vi "FLL Tournament Display Double Qualifier.vi"() -> ()   [LabVIEW 2013]
uses:
  Team_List_Ctrl.ctl
  Team_Scores_And_Rankings_Array_Ctrl.ctl
  Round_And_Score_Ctrl.ctl
  Timer_Details_Ctrl.ctl
  Sound Info.ctl
  <vilib>/sound2/lvsound2.llb/Sound Data Format.ctl
  <vilib>/sound2/lvsound2.llb/Sampling Mode.ctl
  SponsorImageFreqArray.ctl
  <vilib>/picture/picture.llb/imagedata.ctl
  <vilib>/sound2/lvsound2.llb/Sound Output Set Volume (Single).vi
  <vilib>/sound2/lvsound2.llb/Sound Output Write (DBL).vi
  <vilib>/httpClient/LabVIEWHTTPClient.lvlib
panel:
  out "SFA 2":string[][](array[string])
  out "Full Team List 2":T1[](array[typedef])
  out "Reported Scores and Rankings 2":T2
  out "Consolidated Scores and Rankings 2":T4(array[cluster])
  out "IP Address / Port 2":string
  in  "Hurry-Up Sound Volume":dbl(slide)=88.46153846153847 scale=0.0..100.0
  in  "Pre-Match Coundown Sound Volume":dbl(slide)=88.46153846153847 scale=0.0..100.0
  in  "Uh-Oh Sound Volume":dbl(slide)=88.46153846153847 scale=0.0..100.0
  in  "Stop Sound Volume":dbl(slide)=100.0 scale=0.0..100.0
  in  "Start Sound Volume":dbl(slide)=100.0 scale=0.0..100.0
  out "Sound Cluster 2":T5={"Start"={"total number of samples/ch"=31680, "sound format"={"sample rate (S/s)"=11025.0, "number of channels"=1, "bits per sample"=16}, "data"=[{"t0"=timestamp(0 s since 1904-01-01), "dt"=9.070294784580499e-05, "Y"=array[31680 elements]}], "Volume"=100.0}, "Stop"={"total number of samples/ch"=27648, "sound format"={"sample rate (S/s)"=11025.0, "number of channels"=1, "bits per sample"=16}, "data"=[{"t0"=timestamp(0 s since 1904-01-01), "dt"=9.070294784580499e-05, "Y"=array[27648 elements]}], "Volume"=100.0}, "Uh-Oh"={"total number of samples/ch"=29952, "sound format"={"sample rate (S/s)"=11025.0, "number of channels"=1, "bits per sample"=16}, "data"=[{"t0"=timestamp(0 s since 1904-01-01), "dt"=9.070294784580499e-05, "Y"=array[29952 elements]}], "Volume"=88.46153846153847}, "PreMatch"={"total number of samples/ch"=225792, "sound format"={"sample rate (S/s)"=44100.0, "number of channels"=2, "bits per sample"=16}, "data"=[{"t0"=timestamp(0 s since 1904-01-01), "dt"=2.2675736961451248e-05, "Y"=array[225792 elements]}, {"t0"=timestamp(0 s since 1904-01-01), "dt"=2.2675736961451248e-05, "Y"=array[225792 elements]}], "Volume"=75.38461538461539}, "Hurry-Up"={"total number of samples/ch"=0, "sound format"={"sample rate (S/s)"=0.0, "number of channels"=0, "bits per sample"=0}, "data"=[], "Volume"=0.0}}
  in  "stop":bool
  in  "Sound To Play":T7(ring)
  out "Primary Sound Array":dbl[](array[numeric])
  out "PrePrimary Sound Array":dbl[](array[numeric])
  out "Secondary (s)":dbl
  out "Primary (s)":dbl
  out "Pre-Primary (s)":dbl
  out "Master Volume":dbl
  out "Sound Cluster":T5={"Start"={"total number of samples/ch"=31680, "sound format"={"sample rate (S/s)"=11025.0, "number of channels"=1, "bits per sample"=16}, "data"=[{"t0"=timestamp(0 s since 1904-01-01), "dt"=9.070294784580499e-05, "Y"=array[31680 elements]}], "Volume"=100.0}, "Stop"={"total number of samples/ch"=27648, "sound format"={"sample rate (S/s)"=11025.0, "number of channels"=1, "bits per sample"=16}, "data"=[{"t0"=timestamp(0 s since 1904-01-01), "dt"=9.070294784580499e-05, "Y"=array[27648 elements]}], "Volume"=100.0}, "Uh-Oh"={"total number of samples/ch"=29952, "sound format"={"sample rate (S/s)"=11025.0, "number of channels"=1, "bits per sample"=16}, "data"=[{"t0"=timestamp(0 s since 1904-01-01), "dt"=9.070294784580499e-05, "Y"=array[29952 elements]}], "Volume"=88.46153846153847}, "PreMatch"={"total number of samples/ch"=225792, "sound format"={"sample rate (S/s)"=44100.0, "number of channels"=2, "bits per sample"=16}, "data"=[{"t0"=timestamp(0 s since 1904-01-01), "dt"=2.2675736961451248e-05, "Y"=array[225792 elements]}, {"t0"=timestamp(0 s since 1904-01-01), "dt"=2.2675736961451248e-05, "Y"=array[225792 elements]}], "Volume"=75.38461538461539}, "Hurry-Up"={"total number of samples/ch"=0, "sound format"={"sample rate (S/s)"=0.0, "number of channels"=0, "bits per sample"=0}, "data"=[], "Volume"=0.0}}
  out "EnableSounds":bool
  out "Score Behavior":T8(ring)
  out "SFA":string[][](array[string])
  out "NumRoundsToShow":string
  out "Cancelled?":bool
  out "IP Address / Port":string
  in  "Scores Tab":enum32{"3 Rounds", "4 Rounds"}(tab)
  out "Division 1 String 2":string="TESLA DIVISION"
  in  "Scores Box 3":i32[](listbox)
  out "Division 1 String":string="LOVELACE DIVISION"
  in  "Scores Box":i32[](listbox)
  in  "Scores Box 2":i32(listbox)=3
  in  "Top Tab":enum32{"Page 1"}(tab)
  out "Main Logo Image":picture
  out "Powered By LabVIEW":picture
  out "FIRST LEGO League":picture
  out "Match Indicator":string
  out "Tournament Title String":string="Central Texas FLL - Del Valle Double Qualifier Tournament"
  out "TIMER":string="2 : 3 0"
  out "Top Sponsor Image":picture
  out "Mid Sponsor Image":picture
  out "Bottom Sponsor Image":picture
  out "Timer Properties":T9
  out "Consolidated Scores and Rankings":T4(array[cluster])
  out "Reported Scores and Rankings":T2
  out "Full Team List":T1[](array[typedef])
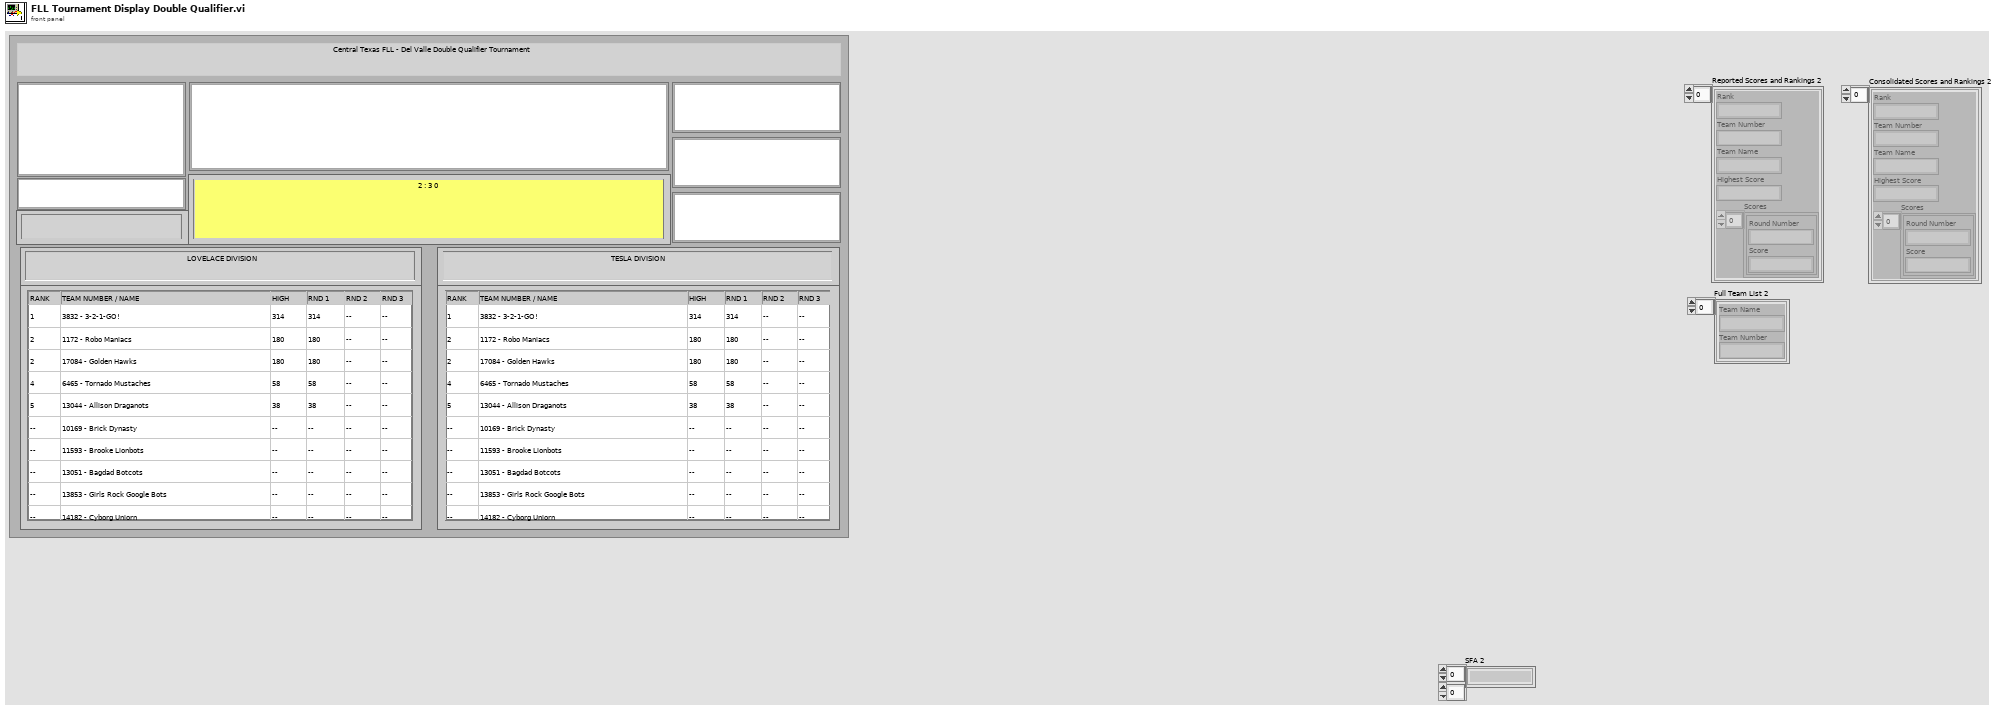
[diagram p1: front panel]
types:
  T1 = typedef "Team_List_Ctrl.ctl" = cluster{"Team Name":string, "Team Number":string}
  T2 = typedef "Team_Scores_And_Rankings_Array_Ctrl.ctl" = cluster{"Rank":string, "Team Number":string, "Team Name":string, "Highest Score":string, "Scores":T3[]}[]
  T3 = typedef "Round_And_Score_Ctrl.ctl" = cluster{"Score":string, "Round Number":string}
  T4 = cluster{"Rank":string, "Team Number":string, "Team Name":string, "Highest Score":string, "Scores":T3[]}[]
  T5 = typedef "Sound Info.ctl" = cluster{"Start":cluster{"total number of samples/ch":u32, "sound format":T6, "data":waveform(dbl)[], "Volume":dbl}, "Stop":cluster{"total number of samples/ch":u32, "sound format":T6, "data":waveform(dbl)[], "Volume":dbl}, "Uh-Oh":cluster{"total number of samples/ch":u32, "sound format":T6, "data":waveform(dbl)[], "Volume":dbl}, "PreMatch":cluster{"total number of samples/ch":u32, "sound format":T6, "data":waveform(dbl)[], "Volume":dbl}, "Hurry-Up":cluster{"total number of samples/ch":u32, "sound format":T6, "data":waveform(dbl)[], "Volume":dbl}}
  T6 = typedef "Sound Data Format.ctl" = cluster{"sample rate (S/s)":dbl, "number of channels":i32, "bits per sample":i32}
  T7 = enum16{"None", "Start", "Stop", "Uh-Oh", "Prematch", "Hurry-Up"}
  T8 = enum16{"Show Negative Scores as ZERO", "Show Negative Scores"}
  T9 = typedef "Timer_Details_Ctrl.ctl" = cluster{"TimeRemaining":string, "MatchPhase":string, "CurrentMatch":string, "Timer_Running":string, "Seconds":string, "LastSound":string}
  T10 = cluster{"Master Volume":dbl, "Pre-Primary (s)":dbl, "Primary (s)":dbl, "Secondary (s)":dbl, "Start Sound Path":path, "Stop Sound Path":path, "Uh-Oh Sound Path":path, "Pre-Match Countdown Sound":path, "Hurry Up Sound":path, "Start Sound Volume":dbl, "Stop Sound Volume":dbl, "Uh-Oh Sound Volume":dbl, "Pre-Match Coundown Sound Volume":dbl, "Hurry Up Sound Volume":dbl}
  T11 = typedef "SponsorImageFreqArray.ctl" = cluster{"Cluster":cluster{"Array":T12[], "Frequency (s)":dbl}, "Cluster":cluster{"Array":T12[], "Frequency (s)":dbl}, "Cluster":cluster{"Array":T12[], "Frequency (s)":dbl}}
  T12 = typedef "imagedata.ctl" = cluster{"image type":i32, "image depth":i32, "image":u8[], "mask":u8[], "colors":u32[], "Rectangle":cluster{"left":i16, "top":i16, "right":i16, "bottom":i16}}
  T13 = typedef "LabVIEWHTTPClient.lvlib/ClientHandle.ctl" = refnum<k1>
  T14 = typedef "Team_List_Array_Ctrl.ctl" = T1[]
  T15 = cluster{"[0]":string, "[1]":string, "[2]":string, "[3]":string}
  T16 = enum32{"Invalid", "Standard", "Closed", "Hidden", "Minimized", "Maximized"}
  T17 = enum32{"invalid app kind", "Development System", "Run Time System", "Student Edition", "Embedded LabVIEW", "Evaluation", "Custom"}
  T18 = cluster{"total number of samples/ch":u32, "sound format":T6, "data":waveform(dbl)[], "Volume":dbl}
  T19 = typedef "Sampling Mode.ctl" = i32
  T20 = typedef "Sound Output Task ID.ctl" = u32
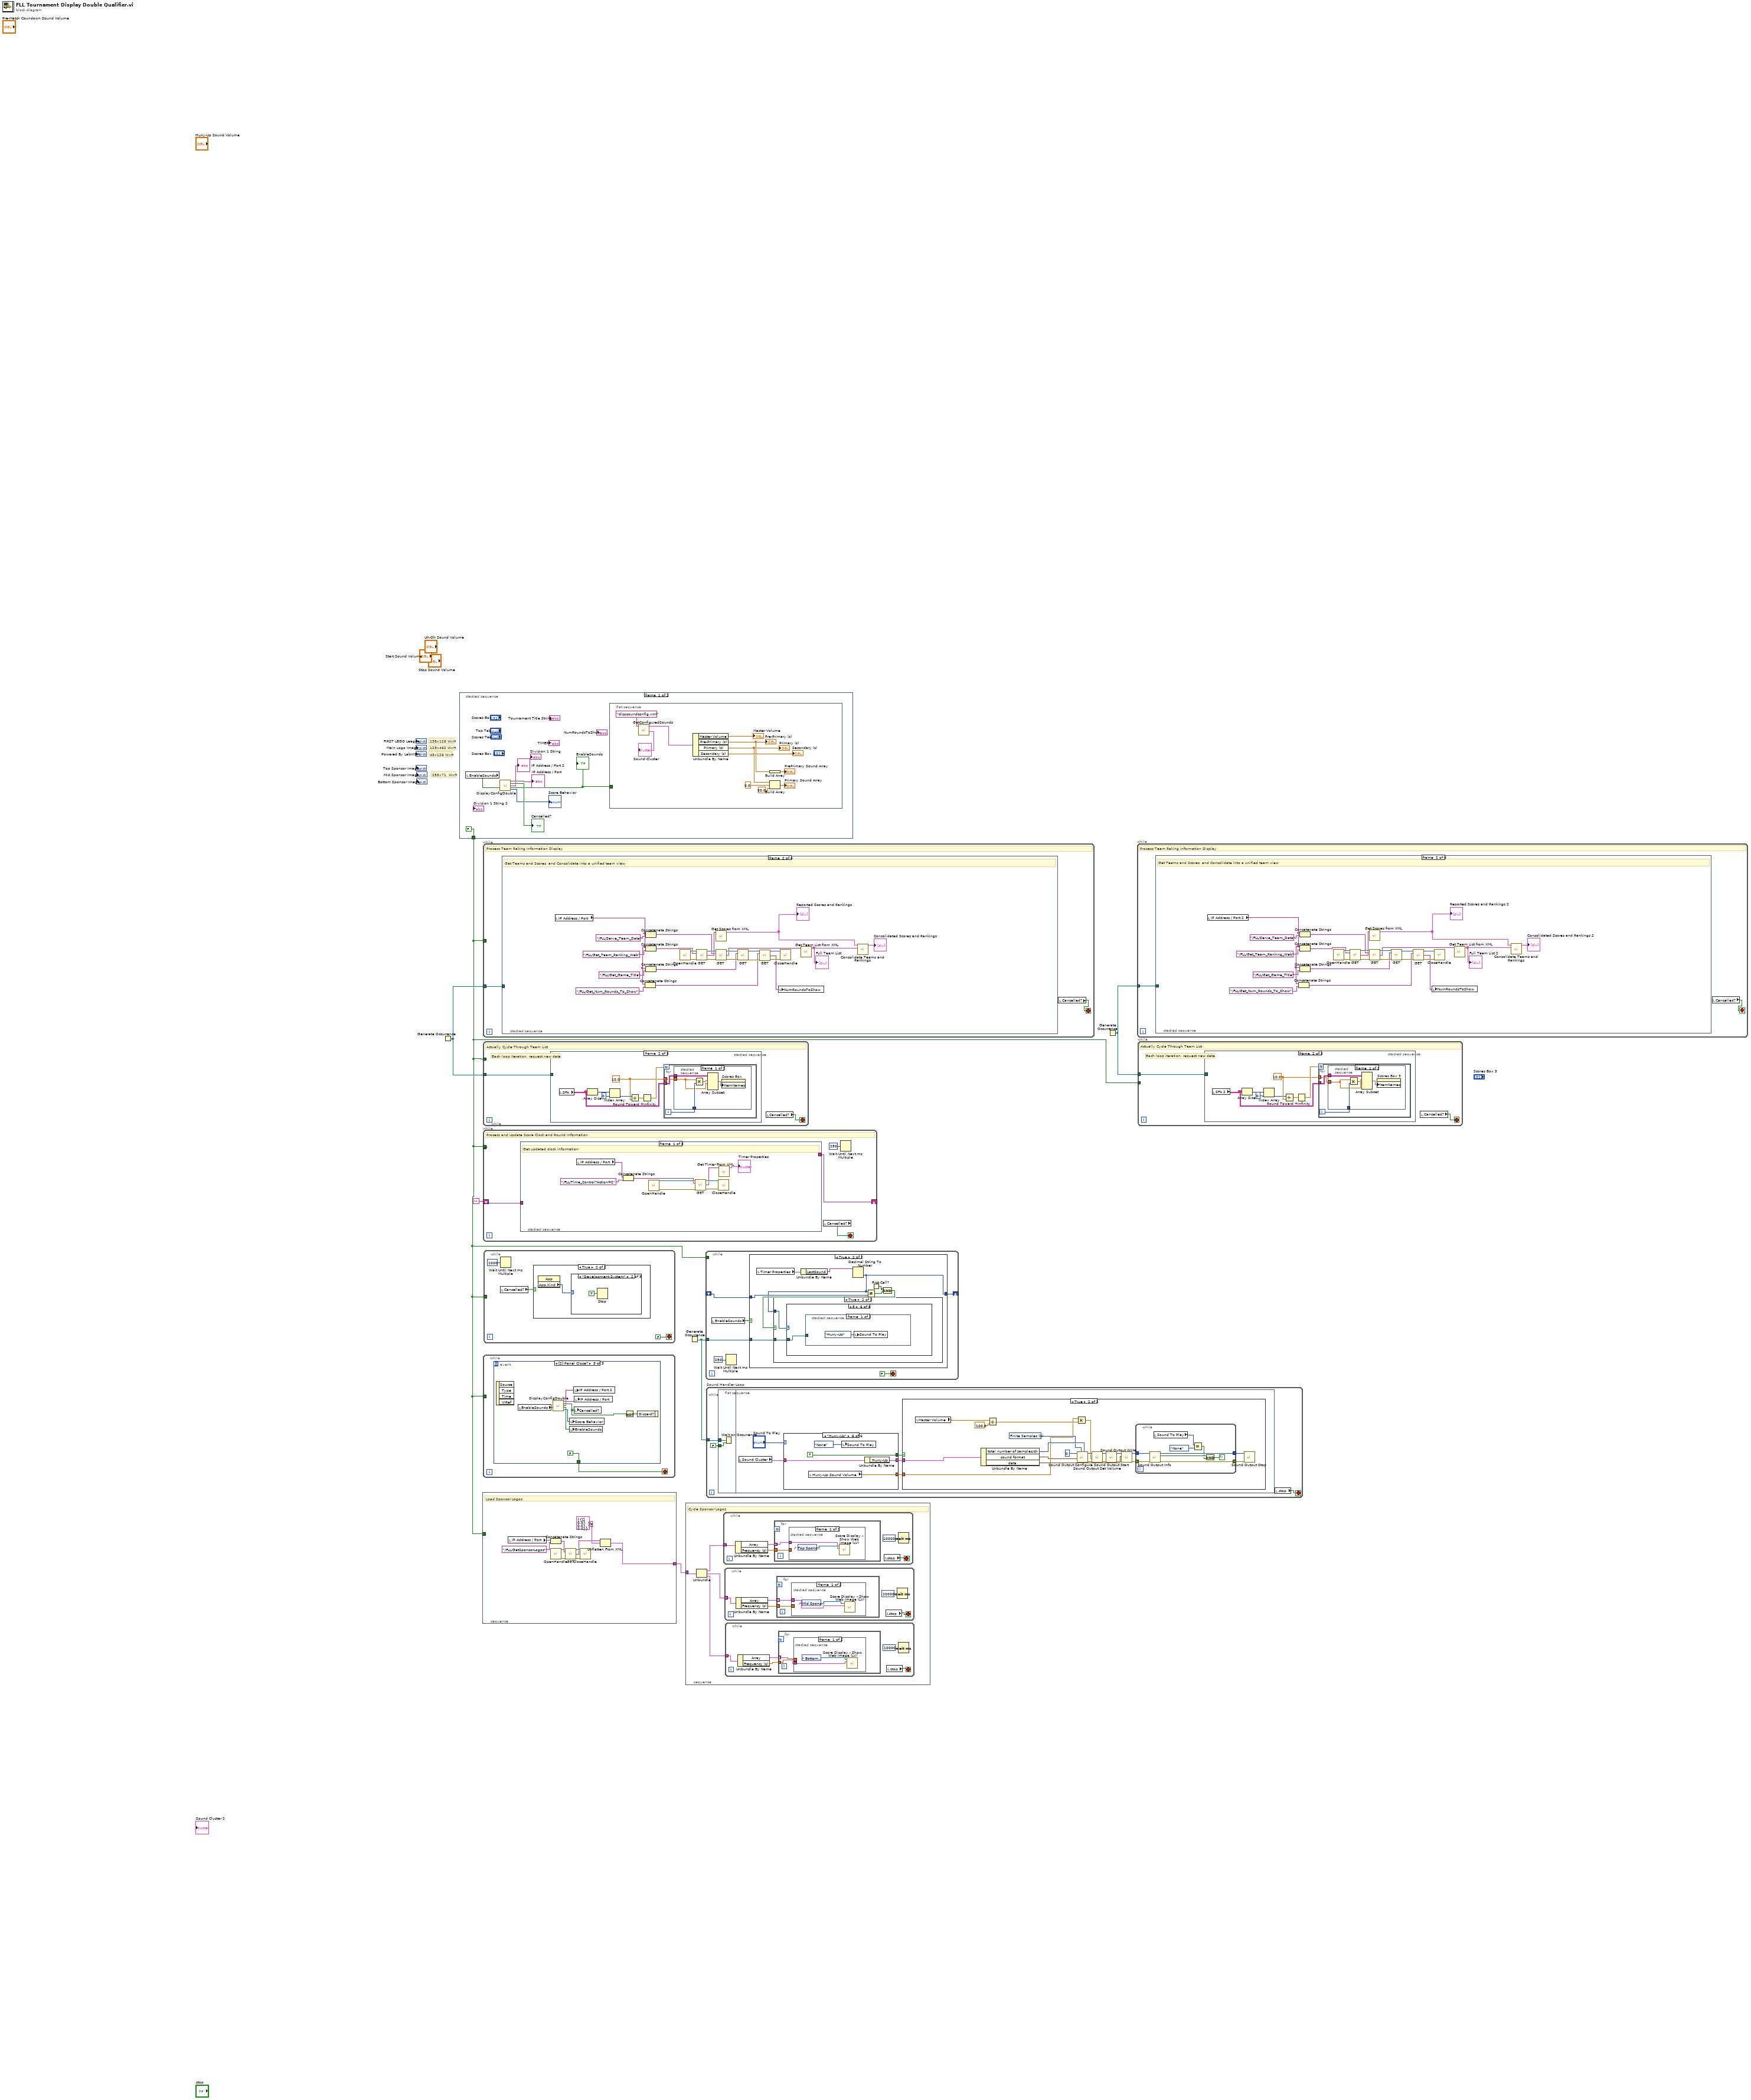
[diagram p0: block diagram]
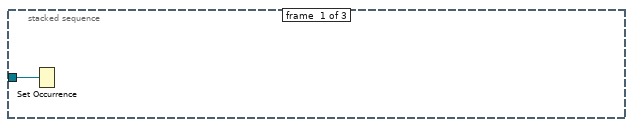
[diagram p2: hidden frame]
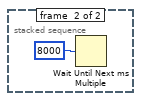
[diagram p3: hidden frame]
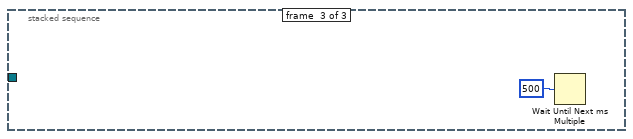
[diagram p4: hidden frame]
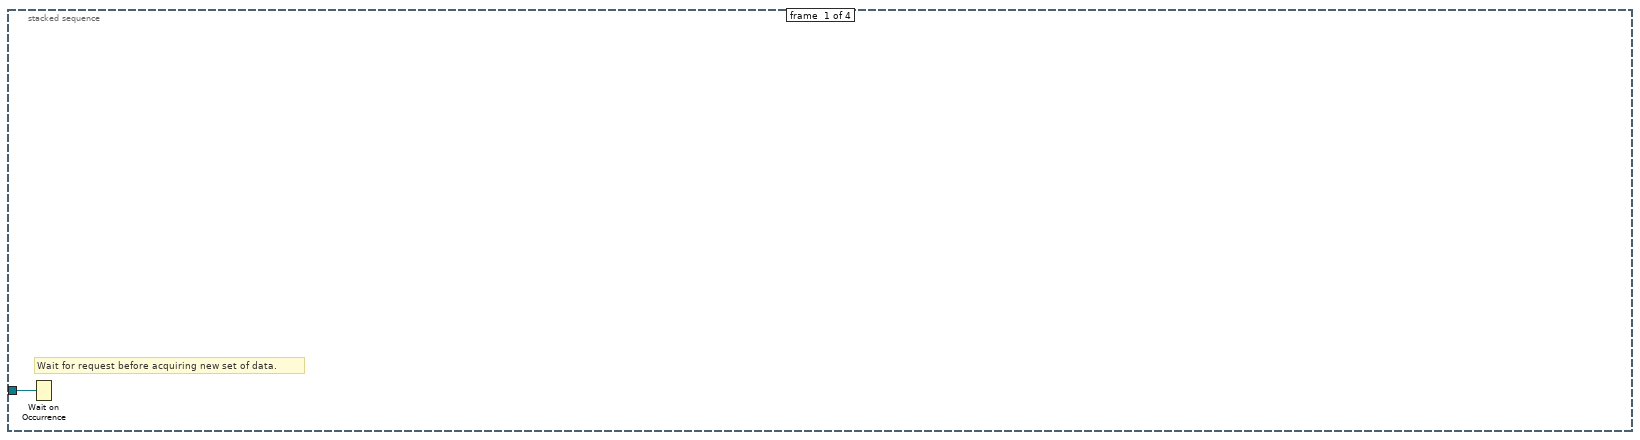
[diagram p5: hidden frame]
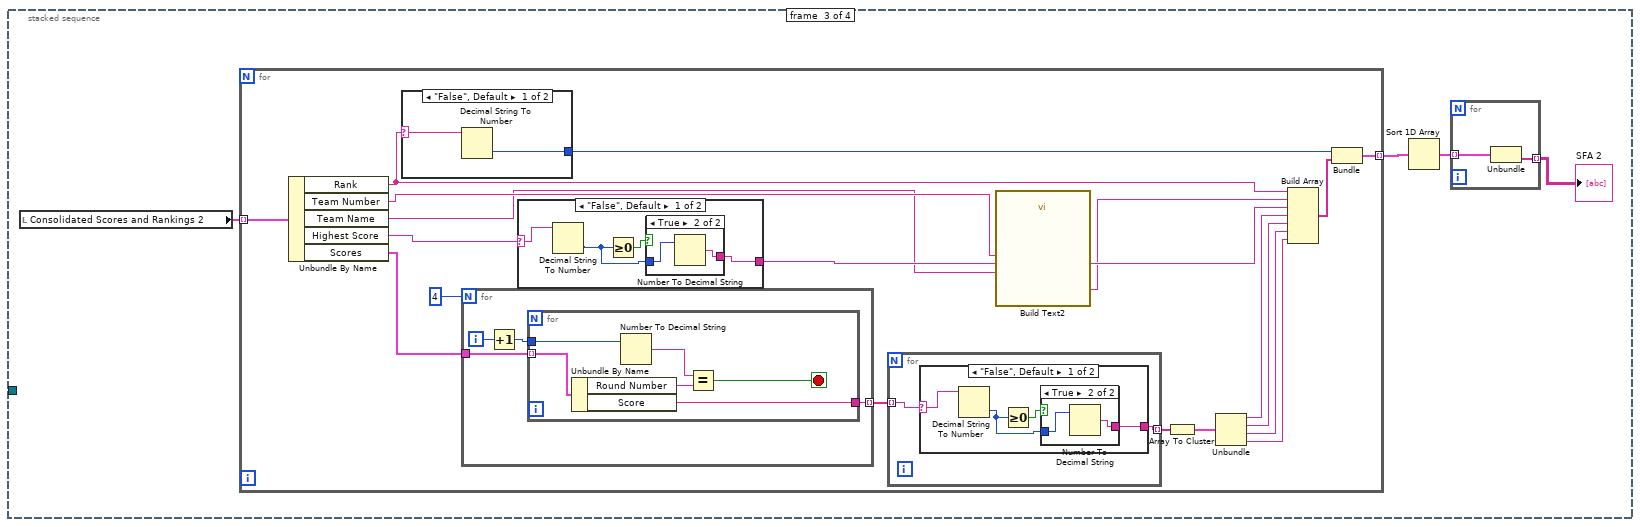
[diagram p6: hidden frame]
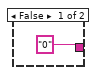
[diagram p7: hidden frame]
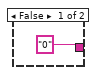
[diagram p9: hidden frame]
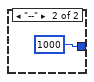
[diagram p11: hidden frame]
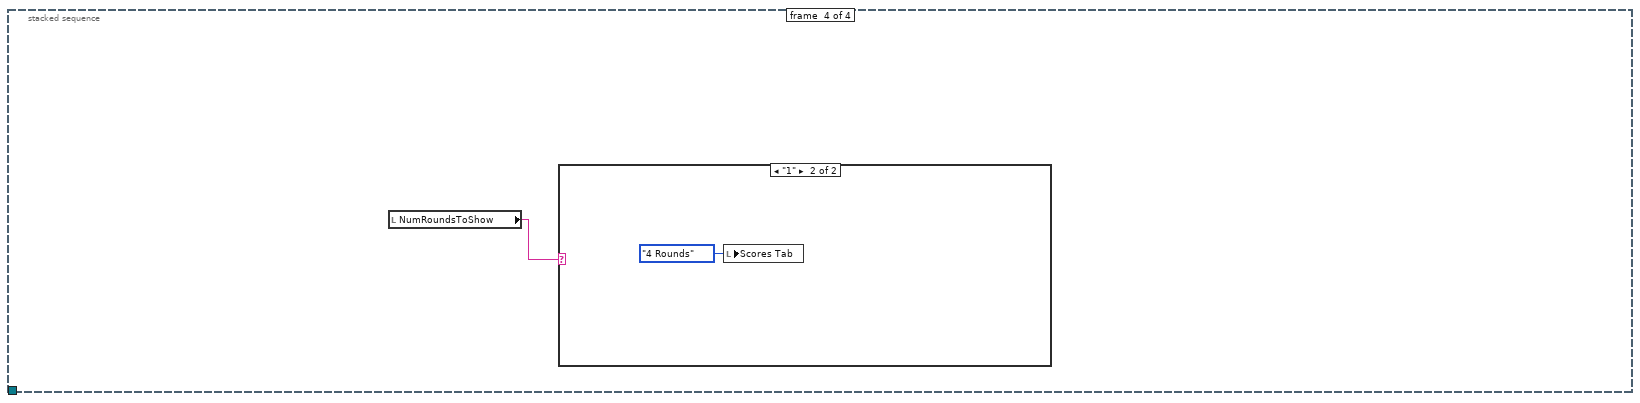
[diagram p12: hidden frame]
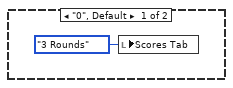
[diagram p13: hidden frame]
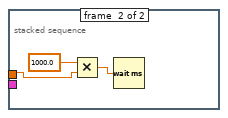
[diagram p14: hidden frame]
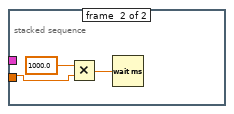
[diagram p15: hidden frame]
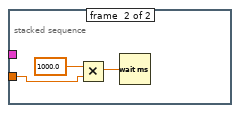
[diagram p16: hidden frame]
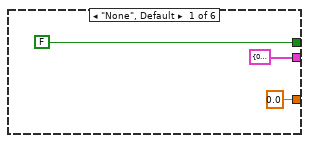
[diagram p18: hidden frame]
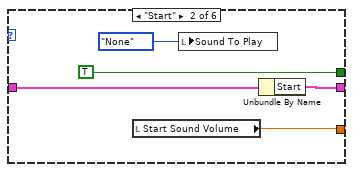
[diagram p19: hidden frame]
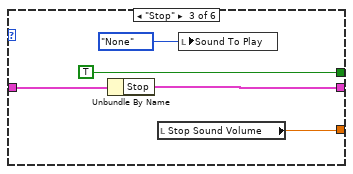
[diagram p20: hidden frame]
diagram:
  # "129x462 WxH"
  # "43x126 WxH"
  # "253x71  WxH"
  # "138x126 WxH"
  n1 = Generate Occurrence() -> (w5:refnum<k4>)
  n2 = stacked-sequence {
    tunnel: [FALSE _] -> w1
    frame #0 {
      n3 = local read "EnableSounds"() -> (w9:bool)
      n4 = call "DisplayConfigDouble.vi"("EnableSounds"=w9) -> ("LovelaceIP"=→"IP Address / Port":string, "Cancelled?"=→"Cancelled?":bool, "TeslaIP"=→"IP Address / Port 2":string, "EnableSounds out"=w8:bool, "Score Behavior OUT"=→"Score Behavior":T8)  [unwired: 10 in]
      "EnableSounds" <- w8
      n5 = flat-sequence {
        tunnel: w8 -> [_]
        frame #0 {
          n6 = call "GetConfiguredSounds.vi"("File"="dispsoundconfig.xml") -> ("Sound Cluster"=→"Sound Cluster":T5, "Settings Cluster"=w23:T10)  [unwired: 9 in]
          n7 = Unbundle By Name(w23) -> ("Master Volume"=→"Master Volume":dbl, "Pre-Primary (s)"=w20:dbl, "Primary (s)"=w18:dbl, "Secondary (s)"=→"Secondary (s)":dbl)
          "Pre-Primary (s)" <- w20
          "Primary (s)" <- w18
          n8 = Build Array(w20) -> (→"PrePrimary Sound Array":dbl[])
          n9 = Build Array(w18, 0.0 ("element"), 30.0 ("element")) -> (→"Primary Sound Array":dbl[])
        }
      }
    }
    frame #1 {
      n10 = disable-structure shown="Disabled" {
        frame Disabled {
          n11 = control-ref of="Powered By LabVIEW"() -> (w29:refnum<vi>)
          n12 = call "Score Display - Auto Scale Image (LV).vi"("Picture Reference"=w29, "path to image file"=path "C:/Users/Danny Diaz/Dropbox/FLL 2 (1).1/Images/powered-by-labview-horiz-logo-rgb.png") -> ()  [unwired: 1 out]
        }
        frame Enabled {
        }
      }
      n13 = disable-structure shown="Disabled" {
        frame Disabled {
          n14 = control-ref of="FIRST LEGO League"() -> (w27:refnum<vi>)
          n15 = call "Score Display - Auto Scale Image (LV).vi"("Picture Reference"=w27, "path to image file"=path "C:/Users/Danny Diaz/Dropbox/FLL 2 (1).1/Images/FLLicon_RGB.jpg") -> ()  [unwired: 1 out]
        }
        frame Enabled {
        }
      }
      n16 = disable-structure shown="Disabled" {
        frame Disabled {
          n17 = control-ref of="Main Logo Image"() -> (w25:refnum<vi>)
          n18 = call "Score Display - Auto Scale Image (LV).vi"("Picture Reference"=w25, "path to image file"=path "C:/Users/Danny Diaz/Dropbox/FLL 2 (1).1/Images/res Fury Logo SM.jpg") -> ()  [unwired: 1 out]
        }
        frame Enabled {
        }
      }
    }
  }
  n19 = stacked-sequence {
    tunnel: w1 -> [_]
    tunnel: [w31] -> w4
    frame #0 {
      # "Load Sponsor Logos"
      n20 = local read "IP Address / Port"() -> (w40:string)
      n21 = Concatenate Strings(w40, "/FLL/GetSponsorLogos" ("url")) -> (w39:string)
      n22 = call <vilib>:"OpenHandle.vi"() -> ("client handle out"=w35:T13, "error out"=w34:errorcluster)  [unwired: 14 in]
      n23 = call <vilib>:"GET.vi"("client handle"=w35, "url"=w39, "error in (no error)"=w34) -> ("client handle out"=w36:T13, "body"=w33:string, "error out"=w37:errorcluster)  [unwired: 9 in, 1 out]
      n24 = call <vilib>:"CloseHandle.vi"("client handle"=w36, "error in (no error)"=w37) -> ()  [unwired: 13 in, 1 out]
      n25 = Unflatten From XML(xml string=w33, type=T11 {"Cluster"={"Array"=[], "Frequency (s)"=0.0}, "Cluster"={"Array"=[], "Frequency (s)"=0.0}, "Cluster"={"Array"=[], "Frequency (s)"=0.0}} ("output cluster")) -> (value=w31:T11)  [unwired: 1 in, 1 out]
    }
  }
  n26 = while {
    tunnel: w1 -> [_]
    tunnel: w5 -> [w41]
    stop <- w42 stop-if-true
    # "Process Team Raking Information Display"
    n27 = stacked-sequence {
      tunnel: w41 -> [w43 _ _ _]
      frame #0 {
        # "Wait for request before acquiring new set of data."
        n28 = Wait on Occurrence(2:w43) -> ()  [unwired: 2 in, 1 out]
      }
      frame #1 {
        # "Get Teams and Scores, and Consolidate into a unified team view"
        n29 = local read "IP Address / Port"() -> (w46:string)
        n30 = Concatenate Strings(w46, "/FLL/Get_Num_Rounds_To_Show" ("url")) -> (w45:string)
        n31 = Concatenate Strings(w46, "/FLL/Serve_Team_Data" ("url")) -> (w59:string)
        n32 = Concatenate Strings(w46, "/FLL/Get_Team_Ranking_Web" ("url")) -> (w57:string)
        n33 = Concatenate Strings(w46, "/FLL/Get_Game_Title" ("url")) -> (w52:string)
        n34 = call <vilib>:"OpenHandle.vi"() -> ("client handle out"=w68:T13, "error out"=w66:errorcluster)  [unwired: 14 in]
        n35 = call <vilib>:"GET.vi"("client handle"=w68, "url"=w57, "error in (no error)"=w66) -> ("client handle out"=w65:T13, "body"=w64:string, "error out"=w67:errorcluster)  [unwired: 9 in, 1 out]
        n36 = call "Get Scores from XML.vi"("XML In"=w64) -> ("Team_Scores_And_Rankings_Array"=w62:T4)  [unwired: 10 in]
        "Reported Scores and Rankings" <- w62
        n37 = call <vilib>:"GET.vi"("client handle"=w65, "url"=w59, "error in (no error)"=w67) -> ("client handle out"=w56:T13, "body"=w54:string, "error out"=w55:errorcluster)  [unwired: 9 in, 1 out]
        n38 = call <vilib>:"GET.vi"("client handle"=w56, "url"=w52, "error in (no error)"=w55) -> ("client handle out"=w48:T13, "error out"=w49:errorcluster)  [unwired: 9 in, 2 out]
        n39 = call <vilib>:"GET.vi"("client handle"=w48, "url"=w45, "error in (no error)"=w49) -> ("client handle out"=w51:T13, "body"=w44:string, "error out"=w50:errorcluster)  [unwired: 9 in, 1 out]
        n40 = local write "NumRoundsToShow"(w44) -> ()
        n41 = call <vilib>:"CloseHandle.vi"("client handle"=w51, "error in (no error)"=w50) -> ()  [unwired: 13 in, 1 out]
        n42 = call "Get Team List from XML.vi"("XML In"=w54) -> ("Team List Array"=w63:T14)  [unwired: 10 in]
        "Full Team List" <- w63
        n43 = call "Consolidate Teams and Rankings.vi"("Team List Array"=w63, "Team_Scores_And_Rankings_Array"=w62) -> ("Consolidated Teams and Rankings"=→"Consolidated Scores and Rankings":T4)  [unwired: 9 in]
      }
      frame #2 {
        n44 = local read "Consolidated Scores and Rankings"() -> (w72:T4)
        n45 = for {
          tunnel: w72 -> [w83] mode=indexing
          tunnel: [w82] -> w70 mode=indexing
          n46 = Unbundle By Name(w83) -> ("Rank"=w85:string, "Team Number"=w77:string, "Team Name"=w76:string, "Highest Score"=w81:string, "Scores"=w93:T3[])
          n47 = case shown="\"False\", Default" w85 {
            selector: w85 -> [w113 _]
            tunnel: [w112 1000] -> w84
            frame "False", Default {
              n48 = Decimal String To Number(string=w113) -> (number=w112:i32)  [unwired: 2 in, 1 out]
            }
            frame "--" {
            }
          }
          n49 = for {
            N: 4 -> [_]
            tunnel: w93 -> [w117]
            tunnel: [w115] -> w79 mode=indexing
            i -> [w118]
            n50 = Increment(x=w118) -> (x+1=w116:i32)
            n51 = for {
              tunnel: w117 -> [w120] mode=indexing
              tunnel: w116 -> [w124]
              tunnel: [w119] -> w115
              stop <- w121 stop-if-true
              n52 = Unbundle By Name(w120) -> ("Round Number"=w123:string, "Score"=w119:string)
              n53 = Number To Decimal String(number=w124) -> (decimal integer string=w122:string)  [unwired: 1 in]
              n54 = Equal?(x=w122, y=w123) -> (x = y?=w121:bool)
            }
          }
          n55 = case shown="\"False\", Default" w81 {
            selector: w81 -> [w107 w111]
            tunnel: [w105 w111] -> w80
            frame "False", Default {
              n56 = Decimal String To Number(string=w107) -> (number=w104:i32)  [unwired: 2 in, 1 out]
              n57 = Greater Or Equal To 0?(x=w104) -> (x >= 0?=w106:bool)
              n58 = case shown="True" w106 {
                tunnel: ["0" w110] -> w105
                tunnel: w104 -> [_ w109]
                frame False {
                }
                frame True {
                  n59 = Number To Decimal String(number=w109) -> (decimal integer string=w110:string)  [unwired: 1 in]
                }
              }
            }
            frame "--" {
            }
          }
          n60 = for {
            tunnel: w79 -> [w95] mode=indexing
            tunnel: [w94] -> w78 mode=indexing
            n61 = case shown="\"False\", Default" w95 {
              selector: w95 -> [w98 w103]
              tunnel: [w99 w103] -> w94
              frame "False", Default {
                n62 = Decimal String To Number(string=w98) -> (number=w96:i32)  [unwired: 2 in, 1 out]
                n63 = Greater Or Equal To 0?(x=w96) -> (x >= 0?=w97:bool)
                n64 = case shown="True" w97 {
                  tunnel: ["0" w102] -> w99
                  tunnel: w96 -> [_ w101]
                  frame False {
                  }
                  frame True {
                    n65 = Number To Decimal String(number=w101) -> (decimal integer string=w102:string)  [unwired: 1 in]
                  }
                }
              }
              frame "--" {
              }
            }
          }
          n66 = call "Build Text"("team_number"=w77, "team_name"=w76) -> ("Result"=w75:string)  [unwired: 12 in, 1 out]
          n67 = Array To Cluster(array=w78) -> (cluster=w91:T15)
          n68 = Unbundle(w91) -> ("[0]"=w90:string, "[1]"=w89:string, "[2]"=w88:string, "[3]"=w87:string)
          n69 = Build Array(w85, w75, w80, w90, w89, w88, w87) -> (w86:string[])
          n70 = Bundle(w84, w86) -> (w82:cluster{i32, string[]})  [unwired: 1 in]
        }
        n71 = Sort 1D Array(array=w70) -> (sorted array=w71:cluster{i32, string[]}[])
        n72 = for {
          tunnel: w71 -> [w74] mode=indexing
          tunnel: [w73] -> w69 mode=indexing
          n73 = Unbundle(w74) -> (w73:string[])  [unwired: 1 out]
        }
        "SFA" <- w69
      }
      frame #3 {
        n74 = local read "NumRoundsToShow"() -> (w125:string)
        n75 = case shown="\"1\"" w125 {
          frame "0", Default {
            n76 = local write "Scores Tab"(enum32{"3 Rounds", "4 Rounds"}."3 Rounds" ("Scores Tab")) -> ()
          }
          frame "1" {
            n77 = local write "Scores Tab"(enum32{"3 Rounds", "4 Rounds"}."4 Rounds" ("Scores Tab")) -> ()
          }
        }
      }
    }
    n78 = local read "Cancelled?"() -> (w42:bool)
  }
  n79 = while {
    tunnel: w1 -> [_]
    tunnel: w5 -> [w128]
    stop <- w129 stop-if-true
    # "Each loop iteration, request new data."
    # "Actually Cycle Through Team List"
    n80 = stacked-sequence {
      tunnel: w128 -> [w130 _ _]
      frame #0 {
        n81 = Set Occurrence(w130) -> ()
      }
      frame #1 {
        w131 = 10.0
        n82 = local read "SFA"() -> (w132:string[][])
        n83 = Array Size(array=w132) -> (size(s)=w136:i32[])
        n84 = Index Array(array=w136, index=0) -> (element=w137:i32)
        n85 = Divide(x=w137, y=w131) -> (x/y=w133:dbl)
        n86 = Round Toward +Infinity(x=w133) -> (ceil(x): smallest int >= x=w134:dbl)
        n87 = for {
          N: w134 -> [_]
          tunnel: w132 -> [w140]
          tunnel: w131 -> [w138]
          i -> [w139]
          n88 = stacked-sequence {
            tunnel: w140 -> [w145 _]
            tunnel: w139 -> [w144 _]
            tunnel: w138 -> [w141 _]
            frame #0 {
              n89 = Multiply(x=w141, y=w144) -> (x*y=w143:dbl)
              n90 = Array Subset(array=w145, index (row)=w143, length (row)=w141) -> (w142:string[][])  [unwired: 2 in]
              n91 = property on="Scores Box" class="MCListbox (strict)"("ItemNames"=w142) -> ()  [unwired: 2 in, 2 out]
            }
            frame #1 {
              n92 = Wait Until Next ms Multiple(millisecond multiple=u32 8000) -> ()  [unwired: 1 out]
            }
          }
        }
      }
      frame #2 {
        n93 = Wait Until Next ms Multiple(millisecond multiple=u32 500) -> ()  [unwired: 1 out]
      }
    }
    n94 = local read "Cancelled?"() -> (w129:bool)
  }
  n95 = while {
    shift-right: [w150] -> _
    shift-left: "" -> [w151]
    tunnel: [w149] -> _
    tunnel: w1 -> [w149]
    stop <- w148 stop-if-true
    # "Process and Update Score Clock and Round Information"
    n96 = stacked-sequence {
      tunnel: w151 -> [_ w165 _]
      tunnel: [_ w164 _] -> w150
      frame #0 {
        # "Get updated clock information"
        n97 = local read "IP Address / Port"() -> (w155:string)
        n98 = Concatenate Strings(w155, "/FLL/Time_Control?Action=2" ("url")) -> (w153:string)
        n99 = call <vilib>:"OpenHandle.vi"() -> ("client handle out"=w160:T13, "error out"=w158:errorcluster)  [unwired: 14 in]
        n100 = call <vilib>:"GET.vi"("client handle"=w160, "url"=w153, "error in (no error)"=w158) -> ("client handle out"=w159:T13, "body"=w156:string, "error out"=w157:errorcluster)  [unwired: 9 in, 1 out]
        n101 = call <vilib>:"CloseHandle.vi"("client handle"=w159, "error in (no error)"=w157) -> ()  [unwired: 13 in, 1 out]
        n102 = call "Get Timer From XML.vi"("body"=w156) -> ("Cluster"=→"Timer Properties":T9)  [unwired: 9 in, 1 out]
      }
      frame #1 {
        n103 = local read "Timer Properties"() -> (w167:T9)
        n104 = local read "Timer Properties"() -> (w163:T9)
        n105 = Unbundle By Name(w167) -> ("TimeRemaining"=w164:string)
        n106 = Unbundle By Name(w163) -> ("MatchPhase"=w162:string)
        n107 = Equal?(x=w164, y=w165) -> (x = y?=w166:bool)
        n108 = case shown="True" w166 {
          tunnel: w164 -> [_ w170]
          tunnel: w162 -> [_ w168]
          frame False {
          }
          frame True {
            n109 = case shown="\"2\"" w168 {
              tunnel: [u32 16514929 u32 11272072 u32 16746633 u32 16774656] -> w169
              frame "3", Default {
              }
              frame "1" {
              }
              frame "2" {
              }
              frame "0" {
              }
            }
            n110 = property on="TIMER" class="Str"("Text.BGColor"=w169) -> ()  [unwired: 2 in, 2 out]
            n111 = local write "TIMER"(w170) -> ()
          }
        }
      }
      frame #2 {
        n112 = local read "Timer Properties"() -> (w179:T9)
        n113 = Unbundle By Name(w179) -> ("CurrentMatch"=w177:string)
        n114 = Concatenate Strings("MATCH", " " ("string"), w177) -> (→"Match Indicator":string)
      }
    }
    n115 = local read "Cancelled?"() -> (w148:bool)
    n116 = Wait Until Next ms Multiple(millisecond multiple=u32 250) -> ()  [unwired: 1 out]
  }
  n117 = while {
    tunnel: w1 -> [_]
    stop <- w180 stop-if-true
    n118 = event shown="[2] Panel Close?" {
      selector: _ -> [_ _ _]
      dyn-events: _ -> [_ _ _]
      timeout: _ -> [_ _ _]
      tunnel: [FALSE _ FALSE] -> w180
      event Timeout {
        n119 = event-data() -> ()  [unwired: 1 in, 2 out]
      }
      event Key Down {
        n120 = event-data() -> ("Char"=w183:i16, "ScanCode"=w182:i16)  [unwired: 1 in, 7 out]
        n121 = case shown="1, Default" w183 {
          tunnel: w182 -> [_ w195 _]
          frame 32 {
            n122 = property class="VI"() -> ("FP.State"=w184:T16)  [unwired: 2 in, 2 out]
            n123 = case shown="\"Invalid\", Default" w184 {
              frame "Invalid", Default {
              }
              frame "Standard" {
                n124 = property class="VI"("FP.State"=T16."Maximized" ("Front Panel Window:State"), "Front Panel.TitleBarVis"=FALSE ("Front Panel Window:Title Bar Visible")) -> ()  [unwired: 2 in, 2 out]
              }
              frame "Closed" {
                n125 = property class="VI"("FP.State"=T16."Standard" ("Front Panel Window:State"), "Front Panel.TitleBarVis"=TRUE ("Front Panel Window:Title Bar Visible")) -> ()  [unwired: 2 in, 2 out]
              }
              frame "Hidden" {
                n126 = property class="VI"("FP.State"=T16."Standard" ("Front Panel Window:State"), "Front Panel.TitleBarVis"=TRUE ("Front Panel Window:Title Bar Visible")) -> ()  [unwired: 2 in, 2 out]
              }
              frame "Minimized" {
                n127 = property class="VI"("FP.State"=T16."Standard" ("Front Panel Window:State"), "Front Panel.TitleBarVis"=TRUE ("Front Panel Window:Title Bar Visible")) -> ()  [unwired: 2 in, 2 out]
              }
              frame "Maximized" {
                n128 = property class="VI"("FP.State"=T16."Standard" ("Front Panel Window:State"), "Front Panel.TitleBarVis"=TRUE ("Front Panel Window:Title Bar Visible")) -> ()  [unwired: 2 in, 2 out]
              }
            }
          }
          frame 1, Default {
            n129 = case shown="1" w195 {
              frame 0, Default {
              }
              frame 1 {
                n130 = local read "EnableSounds"() -> (w198:bool)
                n131 = call "DisplayConfigDouble.vi"("EnableSounds"=w198) -> ("LovelaceIP"=w200:string, "Cancelled?"=w201:bool, "TeslaIP"=w196:string, "EnableSounds out"=w197:bool, "Score Behavior OUT"=w199:T8)  [unwired: 10 in]
                n132 = local write "IP Address / Port"(w200) -> ()
                n133 = local write "IP Address / Port 2"(w196) -> ()
                n134 = local write "Score Behavior"(w199) -> ()
                n135 = local write "EnableSounds"(w197) -> ()
                n136 = local write "Cancelled?"(w201) -> ()
              }
            }
          }
          frame 27 {
            # "Pressed C"
          }
        }
      }
      event Panel Close? {
        n137 = event-data() -> ()  [unwired: 1 in, 4 out]
        n138 = local read "EnableSounds"() -> (w204:bool)
        n139 = call "DisplayConfigDouble.vi"("EnableSounds"=w204) -> ("LovelaceIP"=w209:string, "Cancelled?"=w207:bool, "TeslaIP"=w202:string, "EnableSounds out"=w203:bool, "Score Behavior OUT"=w205:T8)  [unwired: 10 in]
        n140 = local write "Score Behavior"(w205) -> ()
        n141 = local write "EnableSounds"(w203) -> ()
        n142 = local write "IP Address / Port 2"(w202) -> ()
        n143 = local write "Cancelled?"(w207) -> ()
        n144 = local write "IP Address / Port"(w209) -> ()
        n145 = Not(x=w207) -> (.not. x?=w208:bool)
        n146 = event-data("Discard?"=w208) -> ()  [unwired: 1 in, 1 out]
      }
    }
  }
  n147 = while {
    tunnel: w1 -> [_]
    stop <- FALSE stop-if-true
    n148 = Wait Until Next ms Multiple(millisecond multiple=u32 1000) -> ()  [unwired: 1 out]
    n149 = local read "Cancelled?"() -> (w212:bool)
    n150 = case shown="True" w212 {
      frame False {
      }
      frame True {
        n151 = property class="App"() -> ("App.Kind"=w213:T17)  [unwired: 2 in, 2 out]
        n152 = case shown="\"Development System\"" w213 {
          frame "invalid app kind", Default {
          }
          frame "Development System" {
            n153 = Stop(stop? (T)=TRUE) -> ()
          }
          frame "Run Time System" {
            n154 = Quit LabVIEW(quit? (T)=TRUE ("stop? (T)")) -> ()
          }
        }
      }
    }
  }
  n155 = stacked-sequence {
    tunnel: w4 -> [w219]
    frame #0 {
      # "Cycle Sponsor Logos"
      n156 = Unbundle(w219) -> ("Cluster"=w218:cluster{"Array":T12[], "Frequency (s)":dbl}, "Cluster"=w217:cluster{"Array":T12[], "Frequency (s)":dbl}, "Cluster"=w216:cluster{"Array":T12[], "Frequency (s)":dbl})
      n157 = while {
        tunnel: w218 -> [w247]
        stop <- w248 stop-if-true
        n158 = Unbundle By Name(w247) -> ("Array"=w246:T12[], "Frequency (s)"=w245:dbl)
        n159 = for {
          tunnel: w246 -> [w249] mode=indexing
          tunnel: w245 -> [w250]
          n160 = stacked-sequence {
            tunnel: w250 -> [_ w253]
            tunnel: w249 -> [w251 _]
            frame #0 {
              n161 = control-ref of="Top Sponsor Image"() -> (w252:refnum<vi>)
              n162 = call "Score Display - Show Web Image (LV).vi"("image data"=w251, "Picture in"=w252) -> ()  [unwired: 10 in]
            }
            frame #1 {
              n163 = Multiply(x=1000.0, y=w253) -> (x*y=w254:dbl)
              n164 = Wait (ms)(milliseconds to wait=w254) -> ()  [unwired: 1 out]
            }
          }
        }
        n165 = local read "stop"() -> (w248:bool)
        n166 = Wait (ms)(milliseconds to wait=u32 10000) -> ()  [unwired: 1 out]
      }
      n167 = while {
        tunnel: w217 -> [w235]
        stop <- w236 stop-if-true
        n168 = Unbundle By Name(w235) -> ("Array"=w234:T12[], "Frequency (s)"=w233:dbl)
        n169 = for {
          tunnel: w234 -> [w237] mode=indexing
          tunnel: w233 -> [w238]
          n170 = stacked-sequence {
            tunnel: w238 -> [_ w241]
            tunnel: w237 -> [w239 _]
            frame #0 {
              n171 = control-ref of="Mid Sponsor Image"() -> (w240:refnum<vi>)
              n172 = call "Score Display - Show Web Image (LV).vi"("image data"=w239, "Picture in"=w240) -> ()  [unwired: 10 in]
            }
            frame #1 {
              n173 = Multiply(x=1000.0, y=w241) -> (x*y=w242:dbl)
              n174 = Wait (ms)(milliseconds to wait=w242) -> ()  [unwired: 1 out]
            }
          }
        }
        n175 = local read "stop"() -> (w236:bool)
        n176 = Wait (ms)(milliseconds to wait=u32 10000) -> ()  [unwired: 1 out]
      }
      n177 = while {
        tunnel: w216 -> [w223]
        stop <- w224 stop-if-true
        n178 = Unbundle By Name(w223) -> ("Array"=w222:T12[], "Frequency (s)"=w221:dbl)
        n179 = for {
          tunnel: w222 -> [w225] mode=indexing
          tunnel: w221 -> [w226]
          n180 = stacked-sequence {
            tunnel: w226 -> [_ w229]
            tunnel: w225 -> [w227 _]
            frame #0 {
              n181 = control-ref of="Bottom Sponsor Image"() -> (w228:refnum<vi>)
              n182 = call "Score Display - Show Web Image (LV).vi"("image data"=w227, "Picture in"=w228) -> ()  [unwired: 10 in]
            }
            frame #1 {
              n183 = Multiply(x=1000.0, y=w229) -> (x*y=w230:dbl)
              n184 = Wait (ms)(milliseconds to wait=w230) -> ()  [unwired: 1 out]
            }
          }
        }
        n185 = local read "stop"() -> (w224:bool)
        n186 = Wait (ms)(milliseconds to wait=u32 10000) -> ()  [unwired: 1 out]
      }
    }
  }
  n187 = Generate Occurrence() -> (w3:refnum<k4>)
  n188 = while {
    tunnel: w1 -> [_]
    shift-right: [w258] -> _
    shift-left: _ -> [w257]
    tunnel: w3 -> [w256]
    stop <- FALSE stop-if-true
    n189 = local read "EnableSounds"() -> (w259:bool)
    n190 = Wait Until Next ms Multiple(millisecond multiple=u32 250) -> ()  [unwired: 1 out]
    n191 = case shown="True" w259 {
      tunnel: [0 w266] -> w258
      tunnel: w257 -> [_ w270]
      tunnel: w256 -> [_ w263]
      frame False {
      }
      frame True {
        n192 = local read "Timer Properties"() -> (w265:T9)
        n193 = Unbundle By Name(w265) -> ("LastSound"=w264:string)
        n194 = Decimal String To Number(string=w264) -> (number=w266:i32)  [unwired: 2 in, 1 out]
        n195 = Not Equal?(x=w266, y=w270) -> (x != y?=w268:bool)
        n196 = First Call?() -> (First Call?: T/F=w269:bool)
        n197 = Compound Arithmetic op=AND(invert w269, w268) -> (w267:bool)
        n198 = case shown="True" w267 {
          tunnel: w266 -> [_ w272]
          tunnel: w263 -> [_ w271]
          frame False {
          }
          frame True {
            n199 = case shown="5" w272 {
              tunnel: w271 -> [_ w273 w276 w279 w282 w285]
              frame 0, Default {
              }
              frame 1 {
                n200 = stacked-sequence {
                  tunnel: w273 -> [_ w275]
                  frame #0 {
                    n201 = local write "Sound To Play"(T7."Start" ("Sound To Play")) -> ()
                  }
                  frame #1 {
                    n202 = Set Occurrence(w275) -> ()
                  }
                }
              }
              frame 2 {
                n203 = stacked-sequence {
                  tunnel: w276 -> [_ w278]
                  frame #0 {
                    n204 = local write "Sound To Play"(T7."Stop" ("Sound To Play")) -> ()
                  }
                  frame #1 {
                    n205 = Set Occurrence(w278) -> ()
                  }
                }
              }
              frame 3 {
                n206 = stacked-sequence {
                  tunnel: w279 -> [_ w281]
                  frame #0 {
                    n207 = local write "Sound To Play"(T7."Uh-Oh" ("Sound To Play")) -> ()
                  }
                  frame #1 {
                    n208 = Set Occurrence(w281) -> ()
                  }
                }
              }
              frame 4 {
                n209 = stacked-sequence {
                  tunnel: w282 -> [_ w284]
                  frame #0 {
                    n210 = local write "Sound To Play"(T7."Prematch" ("Sound To Play")) -> ()
                  }
                  frame #1 {
                    n211 = Set Occurrence(w284) -> ()
                  }
                }
              }
              frame 5 {
                n212 = stacked-sequence {
                  tunnel: w285 -> [_ w287]
                  frame #0 {
                    n213 = local write "Sound To Play"(T7."Hurry-Up" ("Sound To Play")) -> ()
                  }
                  frame #1 {
                    n214 = Set Occurrence(w287) -> ()
                  }
                }
              }
            }
          }
        }
      }
    }
  }
  n215 = while "Sound Handler Loop" {
    tunnel: w3 -> [w289]
    stop <- w290 stop-if-true
    n216 = flat-sequence {
      tunnel: w289 -> [w292]
      tunnel: FALSE ("ignore previous (T)") -> [w291]
      frame #0 {
        n217 = Wait on Occurrence(1:w291, 2:w292) -> ()  [unwired: 1 in, 1 out]
      }
      frame #1 {
        n218 = local read "Sound Cluster"() -> (w296:T5)
        n219 = case shown="\"Hurry-Up\"" "Sound To Play" {
          tunnel: w296 -> [_ w335 w340 w345 w350 w355]
          tunnel: [T18 {"total number of samples/ch"=0, "sound format"={"sample rate (S/s)"=0.0, "number of channels"=0, "bits per sample"=0}, "data"=[], "Volume"=0.0} ("Uh-Oh") w334 w339 w343 w348 w353] -> w295
          tunnel: [FALSE TRUE TRUE TRUE TRUE TRUE] -> w294
          tunnel: [0.0 ("Pre-Match Coundown Sound Volume") w331 w336 w341 w346 w351] -> w293
          frame "None", Default {
          }
          frame "Start" {
            n220 = local read "Start Sound Volume"() -> (w331:dbl)
            n221 = local write "Sound To Play"(enum16{"None", "Start", "Stop", "Uh-Oh"}."None" ("Sound To Play")) -> ()
            n222 = Unbundle By Name(w335) -> ("Start"=w334:T18)
          }
          frame "Stop" {
            n223 = Unbundle By Name(w340) -> ("Stop"=w339:T18)
            n224 = local read "Stop Sound Volume"() -> (w336:dbl)
            n225 = local write "Sound To Play"(enum16{"None", "Start", "Stop", "Uh-Oh"}."None" ("Sound To Play")) -> ()
          }
          frame "Uh-Oh" {
            n226 = local write "Sound To Play"(enum16{"None", "Start", "Stop", "Uh-Oh"}."None" ("Sound To Play")) -> ()
            n227 = local read "Uh-Oh Sound Volume"() -> (w341:dbl)
            n228 = Unbundle By Name(w345) -> ("Uh-Oh"=w343:T18)
          }
          frame "Prematch" {
            n229 = local read "Pre-Match Coundown Sound Volume"() -> (w346:dbl)
            n230 = local write "Sound To Play"(enum16{"None", "Start", "Stop", "Uh-Oh"}."None" ("Sound To Play")) -> ()
            n231 = Unbundle By Name(w350) -> ("PreMatch"=w348:T18)
          }
          frame "Hurry-Up" {
            n232 = local read "Hurry-Up Sound Volume"() -> (w351:dbl)
            n233 = local write "Sound To Play"(enum16{"None", "Start", "Stop", "Uh-Oh"}."None" ("Sound To Play")) -> ()
            n234 = Unbundle By Name(w355) -> ("Hurry-Up"=w353:T18)
          }
        }
        n235 = case shown="True" w294 {
          tunnel: w295 -> [_ w318]
          tunnel: w293 -> [_ w299]
          frame False {
          }
          frame True {
            w316 = T19 0 items=["Finite Samples", "Continuous Samples"] ("sample mode")
            n236 = local read "Master Volume"() -> (w298:dbl)
            n237 = Unbundle By Name(w318) -> ("total number of samples/ch"=w317:u32, "sound format"=w315:T6, "data"=w308:waveform(dbl)[])
            n238 = Divide(x=w298, y=100.0) -> (x/y=w302:dbl)
            n239 = Multiply(x=w299, y=w302) -> (x*y=w301:dbl)
            n240 = call <vilib>:"Sound Output Configure.vi"("number of samples/ch"=w317, "sample mode"=w316, "sound format"=w315, "device ID"=u32 0) -> ("error out"=w313:errorcluster, "task ID"=w314:T20)  [unwired: 6 in]
            n241 = call-poly <vilib>:"Sound Output Set Volume.vi"("error in (no error)"=w313, "volume"=w301, "task ID"=w314) -> ("error out"=w311:errorcluster, "task ID out"=w312:T20)  [unwired: 7 in]
            n242 = call <vilib>:"Sound Output Start.vi"("error in (no error)"=w311, "task ID"=w312) -> ("error out"=w309:errorcluster, "task ID out"=w310:T20)  [unwired: 8 in]
            n243 = call-poly <vilib>:"Sound Output Write.vi"("error in (no error)"=w309, "data"=w308, "task ID"=w310) -> ("error out"=w306:errorcluster, "task ID out"=w307:T20)  [unwired: 7 in]
            n244 = while {
              tunnel: w307 -> [w327]
              tunnel: w306 -> [w326]
              tunnel: [w325] -> w305
              tunnel: [w324] -> w304
              stop <- w319 continue-if-true
              n245 = call <vilib>:"Sound Output Info.vi"("error in (no error)"=w326, "task ID"=w327) -> ("error out"=w324:errorcluster, "is playing?"=w323:bool, "task ID out"=w325:T20)  [unwired: 6 in, 1 out]
              n246 = local read "Sound To Play"() -> (w321:T7)
              n247 = Equal?(x=w321, y=enum16{"None", "Start", "Stop", "Uh-Oh"}."None") -> (x = y?=w322:bool)
              n248 = And(x=w323, y=w322) -> (x .and. y?=w319:bool)
            }
            n249 = call <vilib>:"Sound Output Stop.vi"("error in (no error)"=w304, "task ID"=w305) -> ()  [unwired: 8 in, 2 out]
          }
        }
      }
    }
    n250 = local read "stop"() -> (w290:bool)
  }
  n251 = Generate Occurrence() -> (w2:refnum<k4>)
  n252 = while {
    tunnel: w2 -> [w356]
    stop <- w357 stop-if-true
    # "Process Team Raking Information Display"
    n253 = stacked-sequence {
      tunnel: w356 -> [w358 _ _ _]
      frame #0 {
        # "Wait for request before acquiring new set of data."
        n254 = Wait on Occurrence(2:w358) -> ()  [unwired: 2 in, 1 out]
      }
      frame #1 {
        # "Get Teams and Scores, and Consolidate into a unified team view"
        n255 = local read "IP Address / Port 2"() -> (w361:string)
        n256 = Concatenate Strings(w361, "/FLL/Get_Num_Rounds_To_Show" ("url")) -> (w360:string)
        n257 = Concatenate Strings(w361, "/FLL/Serve_Team_Data" ("url")) -> (w374:string)
        n258 = Concatenate Strings(w361, "/FLL/Get_Team_Ranking_Web" ("url")) -> (w372:string)
        n259 = Concatenate Strings(w361, "/FLL/Get_Game_Title" ("url")) -> (w367:string)
        n260 = call <vilib>:"OpenHandle.vi"() -> ("client handle out"=w383:T13, "error out"=w381:errorcluster)  [unwired: 14 in]
        n261 = call <vilib>:"GET.vi"("client handle"=w383, "url"=w372, "error in (no error)"=w381) -> ("client handle out"=w380:T13, "body"=w379:string, "error out"=w382:errorcluster)  [unwired: 9 in, 1 out]
        n262 = call "Get Scores from XML.vi"("XML In"=w379) -> ("Team_Scores_And_Rankings_Array"=w377:T4)  [unwired: 10 in]
        "Reported Scores and Rankings 2" <- w377
        n263 = call <vilib>:"GET.vi"("client handle"=w380, "url"=w374, "error in (no error)"=w382) -> ("client handle out"=w371:T13, "body"=w369:string, "error out"=w370:errorcluster)  [unwired: 9 in, 1 out]
        n264 = call <vilib>:"GET.vi"("client handle"=w371, "url"=w367, "error in (no error)"=w370) -> ("client handle out"=w363:T13, "error out"=w364:errorcluster)  [unwired: 9 in, 2 out]
        n265 = call <vilib>:"GET.vi"("client handle"=w363, "url"=w360, "error in (no error)"=w364) -> ("client handle out"=w366:T13, "body"=w359:string, "error out"=w365:errorcluster)  [unwired: 9 in, 1 out]
        n266 = local write "NumRoundsToShow"(w359) -> ()
        n267 = call <vilib>:"CloseHandle.vi"("client handle"=w366, "error in (no error)"=w365) -> ()  [unwired: 13 in, 1 out]
        n268 = call "Get Team List from XML.vi"("XML In"=w369) -> ("Team List Array"=w378:T14)  [unwired: 10 in]
        "Full Team List 2" <- w378
        n269 = call "Consolidate Teams and Rankings.vi"("Team List Array"=w378, "Team_Scores_And_Rankings_Array"=w377) -> ("Consolidated Teams and Rankings"=→"Consolidated Scores and Rankings 2":T4)  [unwired: 9 in]
      }
      frame #2 {
        n270 = local read "Consolidated Scores and Rankings 2"() -> (w387:T4)
        n271 = for {
          tunnel: w387 -> [w398] mode=indexing
          tunnel: [w397] -> w385 mode=indexing
          n272 = Unbundle By Name(w398) -> ("Rank"=w400:string, "Team Number"=w392:string, "Team Name"=w391:string, "Highest Score"=w396:string, "Scores"=w408:T3[])
          n273 = case shown="\"False\", Default" w400 {
            selector: w400 -> [w428 _]
            tunnel: [w427 1000] -> w399
            frame "False", Default {
              n274 = Decimal String To Number(string=w428) -> (number=w427:i32)  [unwired: 2 in, 1 out]
            }
            frame "--" {
            }
          }
          n275 = for {
            N: 4 -> [_]
            tunnel: w408 -> [w432]
            tunnel: [w430] -> w394 mode=indexing
            i -> [w433]
            n276 = Increment(x=w433) -> (x+1=w431:i32)
            n277 = for {
              tunnel: w432 -> [w435] mode=indexing
              tunnel: w431 -> [w439]
              tunnel: [w434] -> w430
              stop <- w436 stop-if-true
              n278 = Unbundle By Name(w435) -> ("Round Number"=w438:string, "Score"=w434:string)
              n279 = Number To Decimal String(number=w439) -> (decimal integer string=w437:string)  [unwired: 1 in]
              n280 = Equal?(x=w437, y=w438) -> (x = y?=w436:bool)
            }
          }
          n281 = case shown="\"False\", Default" w396 {
            selector: w396 -> [w422 w426]
            tunnel: [w420 w426] -> w395
            frame "False", Default {
              n282 = Decimal String To Number(string=w422) -> (number=w419:i32)  [unwired: 2 in, 1 out]
              n283 = Greater Or Equal To 0?(x=w419) -> (x >= 0?=w421:bool)
              n284 = case shown="True" w421 {
                tunnel: ["0" w425] -> w420
                tunnel: w419 -> [_ w424]
                frame False {
                }
                frame True {
                  n285 = Number To Decimal String(number=w424) -> (decimal integer string=w425:string)  [unwired: 1 in]
                }
              }
            }
            frame "--" {
            }
          }
          n286 = for {
            tunnel: w394 -> [w410] mode=indexing
            tunnel: [w409] -> w393 mode=indexing
            n287 = case shown="\"False\", Default" w410 {
              selector: w410 -> [w413 w418]
              tunnel: [w414 w418] -> w409
              frame "False", Default {
                n288 = Decimal String To Number(string=w413) -> (number=w411:i32)  [unwired: 2 in, 1 out]
                n289 = Greater Or Equal To 0?(x=w411) -> (x >= 0?=w412:bool)
                n290 = case shown="True" w412 {
                  tunnel: ["0" w417] -> w414
                  tunnel: w411 -> [_ w416]
                  frame False {
                  }
                  frame True {
                    n291 = Number To Decimal String(number=w416) -> (decimal integer string=w417:string)  [unwired: 1 in]
                  }
                }
              }
              frame "--" {
              }
            }
          }
          n292 = call "Build Text2"("team_number"=w392, "team_name"=w391) -> ("Result"=w390:string)  [unwired: 12 in, 1 out]
          n293 = Array To Cluster(array=w393) -> (cluster=w406:T15)
          n294 = Unbundle(w406) -> ("[0]"=w405:string, "[1]"=w404:string, "[2]"=w403:string, "[3]"=w402:string)
          n295 = Build Array(w400, w390, w395, w405, w404, w403, w402) -> (w401:string[])
          n296 = Bundle(w399, w401) -> (w397:cluster{i32, string[]})  [unwired: 1 in]
        }
        n297 = Sort 1D Array(array=w385) -> (sorted array=w386:cluster{i32, string[]}[])
        n298 = for {
          tunnel: w386 -> [w389] mode=indexing
          tunnel: [w388] -> w384 mode=indexing
          n299 = Unbundle(w389) -> (w388:string[])  [unwired: 1 out]
        }
        "SFA 2" <- w384
      }
      frame #3 {
        n300 = local read "NumRoundsToShow"() -> (w440:string)
        n301 = case shown="\"1\"" w440 {
          frame "0", Default {
            n302 = local write "Scores Tab"(enum32{"3 Rounds", "4 Rounds"}."3 Rounds" ("Scores Tab")) -> ()
          }
          frame "1" {
            n303 = local write "Scores Tab"(enum32{"3 Rounds", "4 Rounds"}."4 Rounds" ("Scores Tab")) -> ()
          }
        }
      }
    }
    n304 = local read "Cancelled?"() -> (w357:bool)
  }
  n305 = while {
    tunnel: w2 -> [w443]
    tunnel: w1 -> [_]
    stop <- w444 stop-if-true
    # "Each loop iteration, request new data."
    # "Actually Cycle Through Team List"
    n306 = stacked-sequence {
      tunnel: w443 -> [w445 _ _]
      frame #0 {
        n307 = Set Occurrence(w445) -> ()
      }
      frame #1 {
        w446 = 10.0
        n308 = local read "SFA 2"() -> (w447:string[][])
        n309 = Array Size(array=w447) -> (size(s)=w451:i32[])
        n310 = Index Array(array=w451, index=0) -> (element=w452:i32)
        n311 = Divide(x=w452, y=w446) -> (x/y=w448:dbl)
        n312 = Round Toward +Infinity(x=w448) -> (ceil(x): smallest int >= x=w449:dbl)
        n313 = for {
          N: w449 -> [_]
          tunnel: w447 -> [w455]
          tunnel: w446 -> [w453]
          i -> [w454]
          n314 = stacked-sequence {
            tunnel: w455 -> [w460 _]
            tunnel: w454 -> [w459 _]
            tunnel: w453 -> [w456 _]
            frame #0 {
              n315 = Multiply(x=w456, y=w459) -> (x*y=w458:dbl)
              n316 = Array Subset(array=w460, index (row)=w458, length (row)=w456) -> (w457:string[][])  [unwired: 2 in]
              n317 = property on="Scores Box 3" class="MCListbox (strict)"("ItemNames"=w457) -> ()  [unwired: 2 in, 2 out]
            }
            frame #1 {
              n318 = Wait Until Next ms Multiple(millisecond multiple=u32 8000) -> ()  [unwired: 1 out]
            }
          }
        }
      }
      frame #2 {
        n319 = Wait Until Next ms Multiple(millisecond multiple=u32 500) -> ()  [unwired: 1 out]
      }
    }
    n320 = local read "Cancelled?"() -> (w444:bool)
  }
